vi "read stage.vi"(7 "Combo Box":string(combo)) -> (2 "pos":dbl)   [LabVIEW 2015]
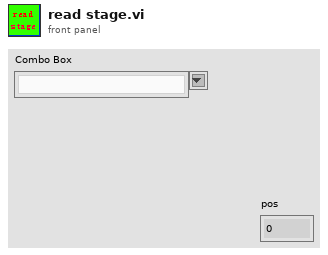
[diagram p1: front panel]
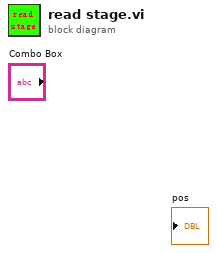
[diagram p0: block diagram]
diagram:
